vi "dvp Vi Set Rgb Gain State.vi"(10 "state":i32, 11 "handle":u32) -> (3 "function return":u32(ring))   [LabVIEW 2018, in "LabViewDVPCamera.lvlib"]
doc: "LabviewDvp2Api dvpStatus dvpViSetRgbGainState(dvpHandle handle, BOOL state);"
uses:
  LabViewDVPCamera.lvlib
  LabViewDVPCamera/LabViewDVPCamera.dll
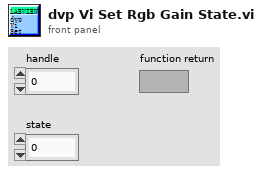
[diagram p1: front panel]
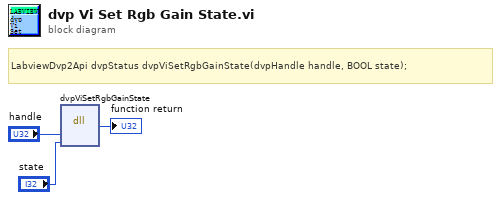
[diagram p0: block diagram]
diagram:
  # "LabviewDvp2Api dvpStatus dvpViSetRgbGainState(dvpHandle handle, BOOL state);"
  n1 = dll-call lib="C:/Program Files (x86)/DVP2 Labview cn 64/Sample/LabViewDVPCamera/LabViewDVPCamera.*" fn="dvpViSetRgbGainState"("handle"="handle", "state"="state") -> (→"function return":u32)  [unwired: 5 in, 2 out]
